vi "gds_rx_config.vi"(0 "Modulation Parameters":T1, 5 "HW parameters In":T2={"Device IP Address"="192.168.11.6", "Active Antenna"="RX1", "Carrier Frequency (Hz)"=915000000.0, "Gain (dB)"=10.0, "Trigger Level"=0.01, "Bandwidth (Hz)"=40000000.0, "Reference Position (%)"=10.0, "Capture Time (s)"=0.0004, "Simulate"=FALSE} {"Capture Time (s)" format="%.2p"; "Bandwidth (Hz)" format="%.2p"; "Trigger Level" format="%#.3p"; "Gain (dB)" format="%.2f"; "Carrier Frequency (Hz)" format="%.2p"}, 11 "error in (no error)":errorcluster) -> (1 "coerced bandwidth":dbl, 2 "coerced carrier frequency (Hz)":dbl=100000.0 format="%#_6p", 3 "coerced gain (dB)":dbl format="%#_6f", 4 "Modulation Parameters Out":T1, 6 "HW parameters Out":T2={"Device IP Address"="192.168.11.6", "Active Antenna"="RX1", "Carrier Frequency (Hz)"=915000000.0, "Gain (dB)"=10.0, "Trigger Level"=0.01, "Bandwidth (Hz)"=40000000.0, "Reference Position (%)"=10.0, "Capture Time (s)"=0.0004, "Simulate"=FALSE} {"Capture Time (s)" format="%.2p"; "Bandwidth (Hz)" format="%.2p"; "Trigger Level" format="%#.3p"; "Gain (dB)" format="%.2f"; "Carrier Frequency (Hz)" format="%.2p"}, 8 "Simulate":bool, 15 "error out":errorcluster)   [LabVIEW 2012]
uses:
  EE 497/LABS/SDR/control_type_defs.llb/rx_hw params.ctl
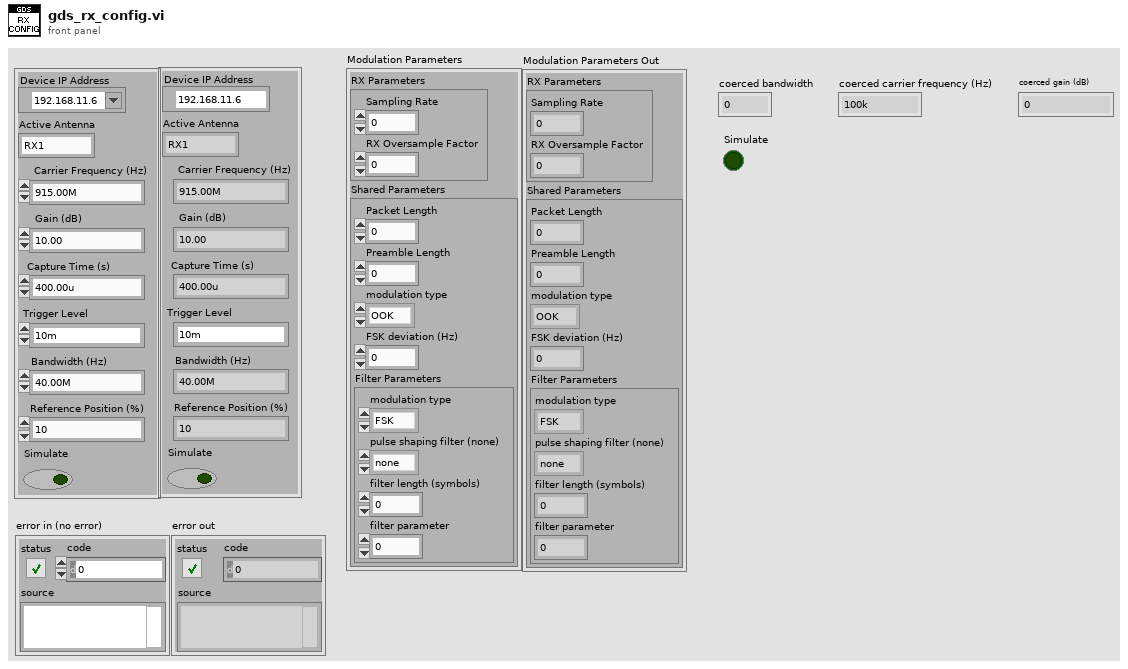
[diagram p1: front panel]
types:
  T1 = cluster{"RX Parameters":cluster{"Sampling Rate":dbl, "RX Oversample Factor":i32}, "Shared Parameters":cluster{"Packet Length":i32, "Preamble Length":i32, "modulation type":enum16{"OOK", "FSK", "PSK", "QAM", "MSK", "PAM", "ASK", "CPM"}, "FSK deviation (Hz)":dbl, "Filter Parameters":cluster{"modulation type":enum16{"FSK", "PSK", "QAM", "MSK", "PAM", "ASK", "CPM"}, "pulse shaping filter (none)":enum16{"none", "Raised Cosine", "Root Raised Cos", "Gaussian"}, "filter length (symbols)":i32, "filter parameter":dbl}}}
  T2 = typedef "rx_hw params.ctl" = cluster{"Device IP Address":refnum<k15>, "Active Antenna":string, "Carrier Frequency (Hz)":dbl, "Gain (dB)":dbl, "Trigger Level":dbl, "Bandwidth (Hz)":dbl, "Reference Position (%)":dbl, "Capture Time (s)":dbl, "Simulate":bool}
  T3 = cluster{"Sampling Rate":dbl, "RX Oversample Factor":i32}
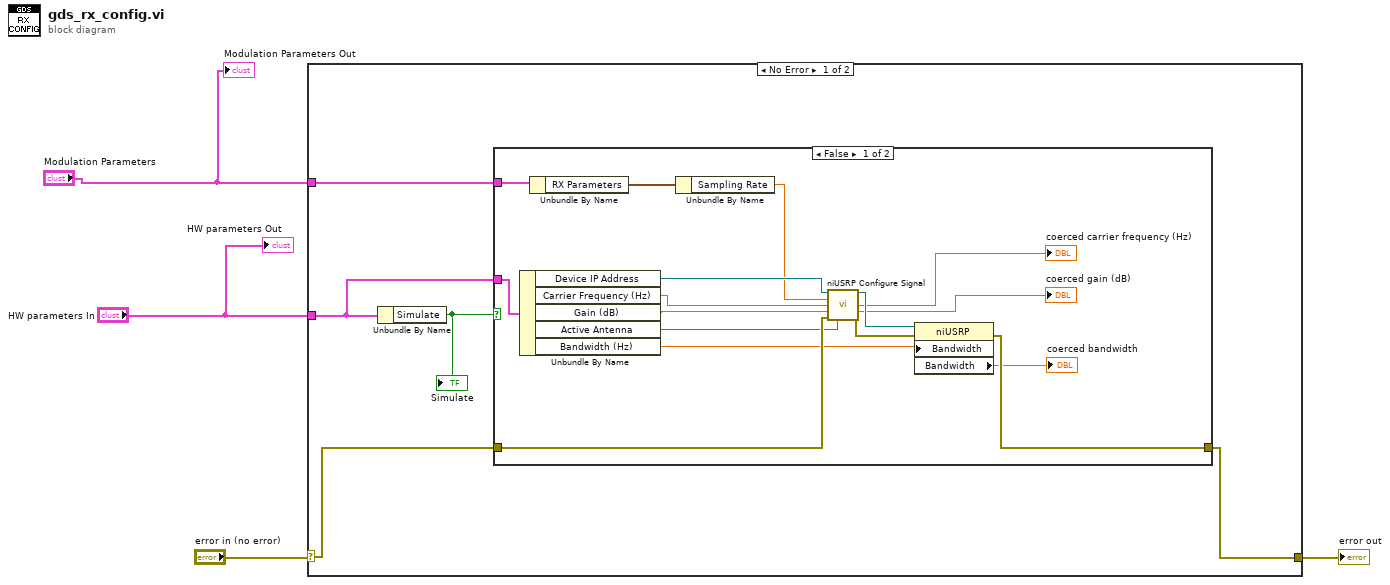
[diagram p0: block diagram]
diagram:
  n1 = case shown="No Error" "error in (no error)" {
    selector: "error in (no error)" -> [w9 w27]
    tunnel: [w8 w27] -> w3
    tunnel: "HW parameters In" -> [w7 _]
    tunnel: "Modulation Parameters" -> [w6 _]
    frame No Error {
      n2 = Unbundle By Name(w7) -> ("Simulate"=w5:bool)
      "Simulate" <- w5
      n3 = case shown="False" w5 {
        tunnel: w9 -> [w20 w26]
        tunnel: [w13 w26] -> w8
        tunnel: w7 -> [w23 _]
        tunnel: w6 -> [w25 _]
        frame False {
          n4 = Unbundle By Name(w23) -> ("Device IP Address"=w22:refnum<k15>, "Carrier Frequency (Hz)"=w19:dbl, "Gain (dB)"=w18:dbl, "Active Antenna"=w17:string, "Bandwidth (Hz)"=w14:dbl)
          n5 = Unbundle By Name(w25) -> ("RX Parameters"=w24:T3)
          n6 = Unbundle By Name(w24) -> ("Sampling Rate"=w21:dbl)
          n7 = call <instrlib>:"niUSRP Configure Signal.vi"("session handle"=w22, "IQ rate"=w21, "carrier frequency"=w19, "gain"=w18, "error in (no error)"=w20, "active antenna"=w17) -> ("session handle out"=w16:refnum<k15>, "coerced carrier frequency"=→"coerced carrier frequency (Hz)":dbl, "coerced gain"=→"coerced gain (dB)":dbl, "error out"=w15:errorcluster)  [unwired: 5 in, 1 out]
          n8 = property class="niUSRP"(reference=w16, error in=w15, "Bandwidth"=w14) -> (error out=w13:errorcluster, "Bandwidth"=→"coerced bandwidth":dbl)  [unwired: 1 out]
        }
        frame True {
        }
      }
    }
    frame Error {
    }
  }
  "error out" <- w3
  "HW parameters Out" <- "HW parameters In"
  "Modulation Parameters Out" <- "Modulation Parameters"
